vi "Define Parameter.vi"(8 "error in (no error)":errorcluster, 11 "Analyze SHG-AK in":refnum<class "Analyze SHG-AK.lvclass">) -> (0 "error out":errorcluster, 3 "Analyze SHG-AK out":refnum<class "Analyze SHG-AK.lvclass">)   [LabVIEW 2020, in "Analyze.lvlib" / "Analyze SHG-AK.lvclass"]
uses:
  Analyze SHG-AK.lvclass
  Analyze BaseClass/Analyze BaseClass/Analyze BaseClass.lvclass
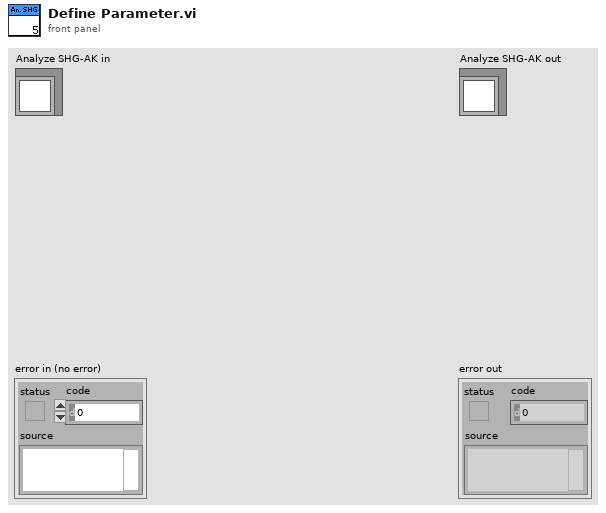
[diagram p1: front panel]
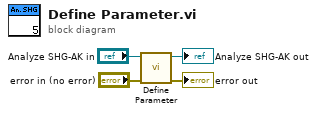
[diagram p0: block diagram]
diagram:
  n1 = call-parent "Define Parameter.vi"("error in (no error)"="error in (no error)", "Analyze BaseClass in"="Analyze SHG-AK in") -> ("error out"=→"error out":errorcluster, "Analyze BaseClass out"=→"Analyze SHG-AK out":refnum<class "Analyze SHG-AK.lvclass">)  [unwired: 8 in]
